vi "Import Sensor Metadata.vi"(10 "Table Strings In":string[][](array[string])=[["Control/Sensors/L1_XBack", "inches", "1.0", "1.0", "<None>", ""], ["Control/Sensors/L1_XFront", "inches", "1.0", "1.0", "<None>", ""], ["Control/Sensors/L1_Y", "inches", "1.0", "1.0", "<None>", ""], ["Control/Sensors/L1_ZBack", "inches", "1.0", "1.0", "<None>", ""], ["Control/Sensors/L1_ZFront", "inches", "1.0", "1.0", "<None>", ""], ["Control/Sensors/L1_ZLeft", "inches", "1.0", "1.0", "<None>", ""]]) -> (2 "Table Strings Out":string[][](array[string]), 3 "Canceled":bool=TRUE)   [LabVIEW 2013]
panel:
  in  "Cancel":bool
  in  "Ok":bool
  in  "Text Block":string=",,,,,\n,,,,,\n,,,,,\n,,,,,\n,,,,,\n,,,,,"
  # "Paste comma and linefeed delimited matrix and press OK"
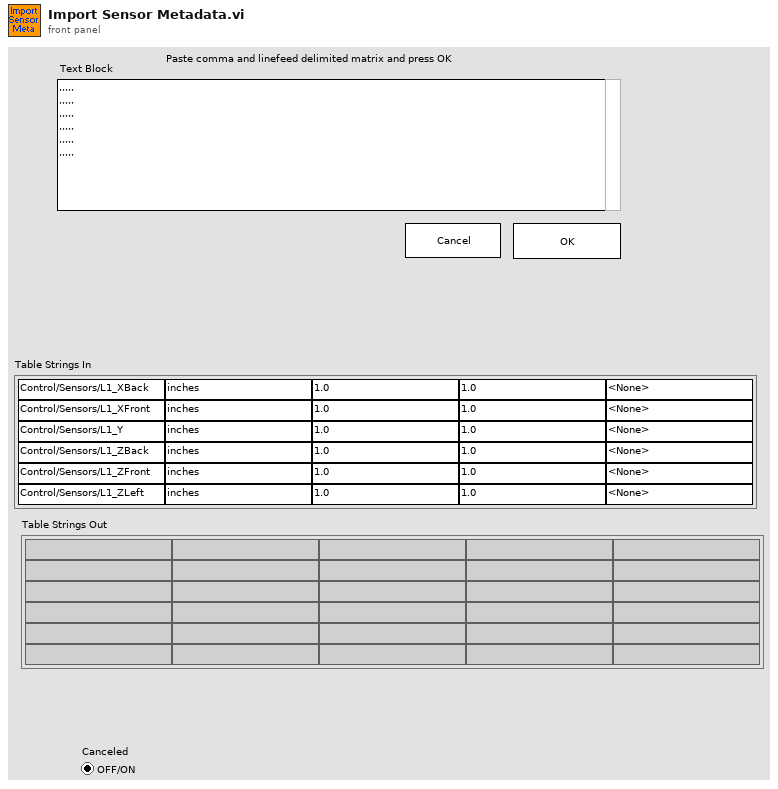
[diagram p1: front panel]
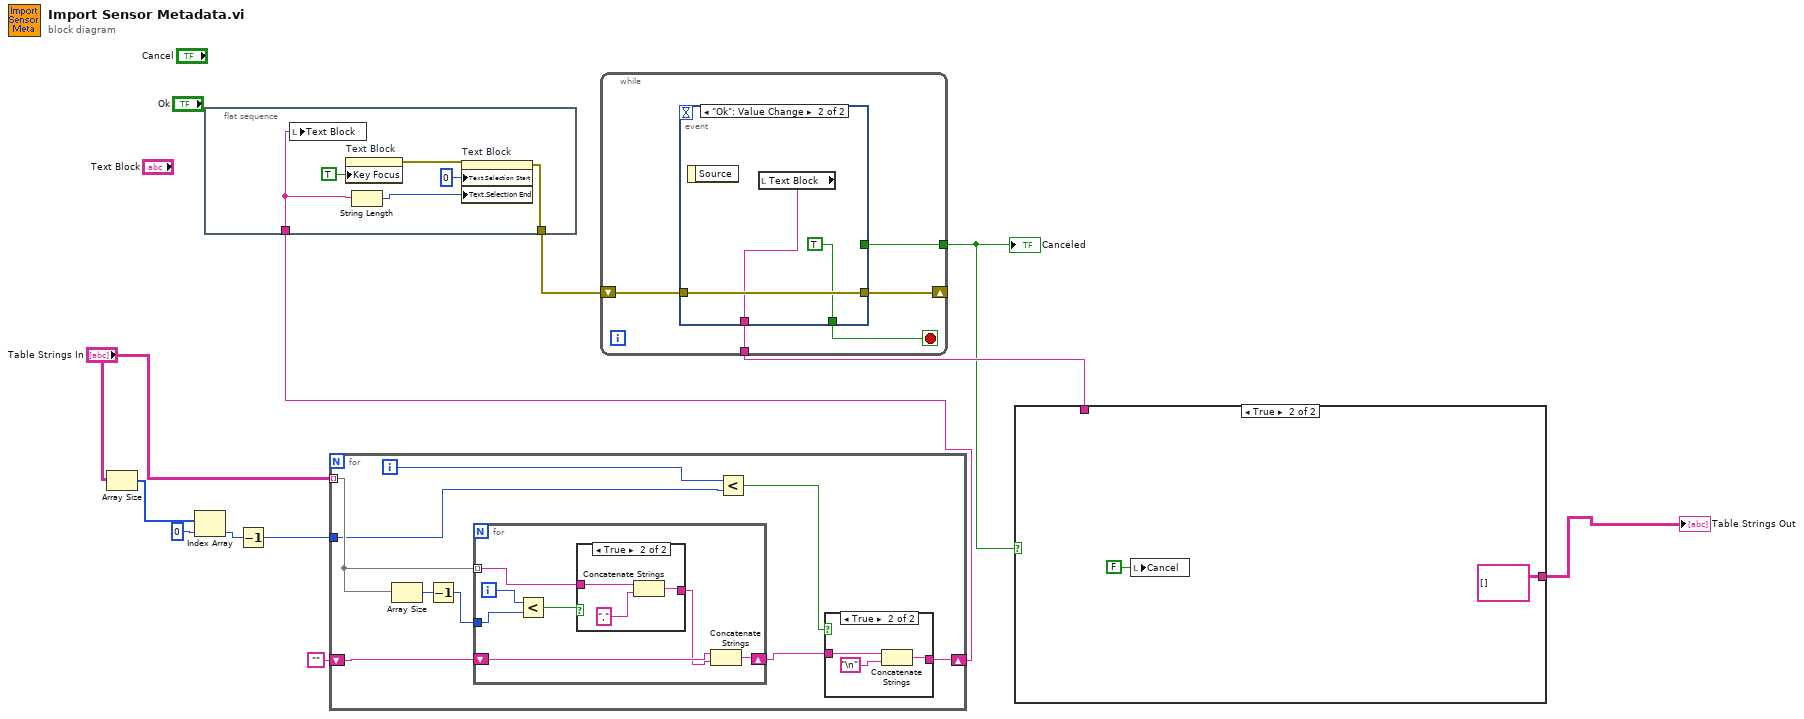
[diagram p0: block diagram]
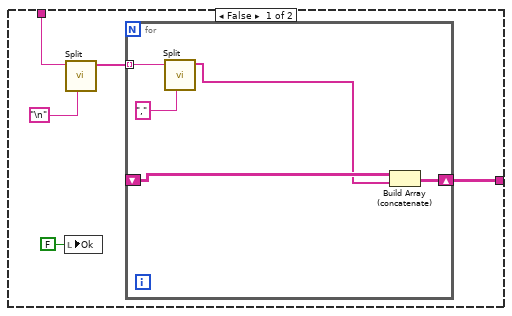
[diagram p4: hidden frame]
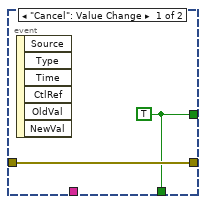
[diagram p5: hidden frame]
diagram:
  n1 = Array Size(array="Table Strings In") -> (size(s)=w8:i32[])
  n2 = Index Array(array=w8, index=0) -> (element=w6:i32)
  n3 = flat-sequence {
    tunnel: [w16] -> w11
    tunnel: w4 -> [w12]
    frame #0 {
      n4 = local write "Text Block"(w12) -> ()
      n5 = property on="Text Block" class="Str"("Key Focus"=TRUE) -> (error out=w14:errorcluster)  [unwired: 2 in, 1 out]
      n6 = String Length(string=w12) -> (length=w13:i32)
      n7 = property on="Text Block" class="Str"(error in=w14, "Text.Selection Start"=u32 0 ("Text.Selection:Start"), "Text.Selection End"=w13) -> (error out=w16:errorcluster)  [unwired: 1 in, 1 out]
    }
  }
  n8 = Decrement(x=w6) -> (x-1=w5:i32)
  n9 = for {
    tunnel: "Table Strings In" -> [w25] mode=indexing
    shift-right: [w18] -> w4
    shift-left: "" -> [w26]
    tunnel: w5 -> [w20]
    i -> [w21]
    n10 = Array Size(array=w25) -> (size(s)=w24:i32)
    n11 = Decrement(x=w24) -> (x-1=w23:i32)
    n12 = for {
      shift-right: [w36] -> w22
      shift-left: w26 -> [w35]
      tunnel: w25 -> [w33] mode=indexing
      tunnel: w23 -> [w31]
      i -> [w32]
      n13 = Less?(x=w32, y=w31) -> (x < y?=w37:bool)
      n14 = case shown="True" w37 {
        tunnel: w33 -> [w38 w41]
        tunnel: [w38 w40] -> w34
        frame False {
        }
        frame True {
          n15 = Concatenate Strings(w41, ",") -> (w40:string)
        }
      }
      n16 = Concatenate Strings(w35, w34) -> (w36:string)
    }
    n17 = Less?(x=w21, y=w20) -> (x < y?=w19:bool)
    n18 = case shown="True" w19 {
      tunnel: w22 -> [w27 w30]
      tunnel: [w27 w28] -> w18
      frame False {
      }
      frame True {
        n19 = Concatenate Strings(w30, "\n") -> (w28:string)
      }
    }
  }
  n20 = while {
    shift-right: [w45] -> _
    shift-left: w11 -> [w46]
    tunnel: [w44] -> w9
    tunnel: [w42] -> w10
    stop <- w43 stop-if-true
    n21 = event shown="[1] \"Ok\": Value Change" {
      selector: _ -> [_ _]
      dyn-events: _ -> [_ _]
      timeout: _ -> [_ _]
      tunnel: w46 -> [w48 w51]
      tunnel: [w48 w51] -> w45
      tunnel: [w47 _] -> w44
      tunnel: [w47 TRUE] -> w43
      tunnel: [_ w49] -> w42
      event "Cancel": Value Change {
        w47 = TRUE
        n22 = event-data() -> ()  [unwired: 1 in, 6 out]
      }
      event "Ok": Value Change {
        n23 = event-data() -> ()  [unwired: 1 in, 1 out]
        n24 = local read "Text Block"() -> (w49:string)
      }
    }
  }
  "Canceled" <- w9
  n25 = case shown="True" w9 {
    tunnel: w10 -> [w56 _]
    tunnel: [w53 string[][] []] -> w1
    frame False {
      n26 = local write "Ok"(FALSE ("Ok")) -> ()
      n27 = call "Split.vi"("delimiter"="\n", "String"=w56) -> ("Array Result"=w54:string[])  [unwired: 9 in]
      n28 = for {
        tunnel: w54 -> [w61] mode=indexing
        shift-right: [w59] -> w53
        shift-left: _ -> [w58]
        n29 = call "Split.vi"("delimiter"=",", "String"=w61) -> ("Array Result"=w57:string[])  [unwired: 9 in]
        n30 = Build Array (concatenate)(w58, w57) -> (w59:string[][])
      }
    }
    frame True {
      n31 = local write "Cancel"(FALSE ("Cancel")) -> ()
    }
  }
  "Table Strings Out" <- w1
